vi "Monitor console and wait for keywords.vi"(6 "VISA resource name":refnum<visa-resource-name>, 7 "Timeout (mSecs)":u32=3000, 8 "error in (no error)":errorcluster, 9 "Wait after":u32=750, 10 "Wait for keywords":string[](array[string])) -> (0 "error out":errorcluster, 1 "Keyword found index":i32, 2 "Response":string, 3 "timeout":bool, 4 "VISA Refnum out":refnum<visa-resource-name>)   [LabVIEW 2024]
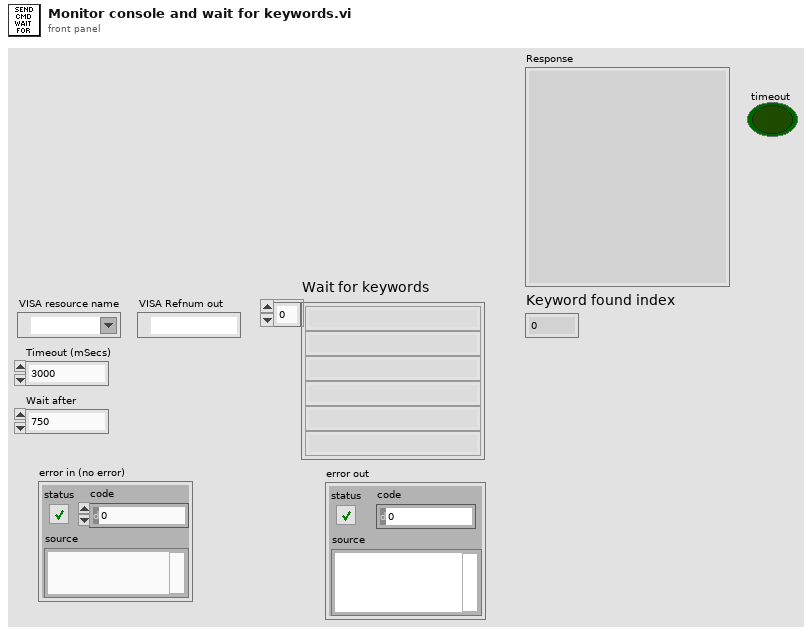
[diagram p1: front panel]
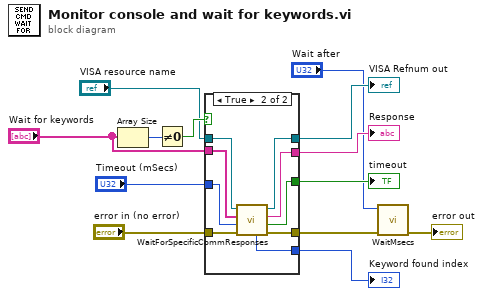
[diagram p0: block diagram]
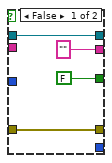
[diagram p2: hidden frame]
diagram:
  n1 = Array Size(array="Wait for keywords") -> (size(s)=w6:i32)
  n2 = Not Equal To 0?(x=w6) -> (x != 0?=w5:bool)
  n3 = case shown="True" w5 {
    tunnel: "VISA resource name" -> [w17 w26]
    tunnel: "error in (no error)" -> [w14 w25]
    tunnel: "Timeout (mSecs)" -> [_ w24]
    tunnel: ["" ("Response") w23] -> w12
    tunnel: [FALSE ("timeout") w22] -> w11
    tunnel: [w17 w21] -> w10
    tunnel: [w14 w20] -> w9
    tunnel: "Wait for keywords" -> [_ w19]
    tunnel: [_ w18] -> w3
    frame False {
    }
    frame True {
      n4 = call "WaitForSpecificCommResponses.vi"("error in (no error)"=w25, "Timeout (mSecs)"=w24, "WaitFor Keywords"=w19, "VISA Refnum in"=w26) -> ("error out"=w20:errorcluster, "timeout"=w22:bool, "Response"=w23:string, "VISA Refnum out"=w21:refnum<visa-resource-name>, "Keyword found index"=w18:i32)  [unwired: 2 in, 1 out]
    }
  }
  "VISA Refnum out" <- w10
  "Response" <- w12
  "timeout" <- w11
  "Keyword found index" <- w3
  n5 = call "WaitMsecs.vi"("error in (no error)"=w9, "Wait Msecs"="Wait after") -> ("error out"=→"error out":errorcluster)  [unwired: 9 in]
